vi "Server - Test Inbound Traffic to Server.vi"(8 "error in (no error)":errorcluster, 10 "client address":string="localhost", 11 "ports to check":u16[](array[numeric])=[82, 482, 5672, 6343, 8002, 49580, 22, 44516, 52725, 8080]) -> (0 "error out":errorcluster, 2 "log file path":path, 3 "Results":string[][](array[string]))   [LabVIEW 2019]
doc: "Demonstrates how to open a connection to an TCP server, read the data being sent, and display the data on a chart. This VI is designed to stop if the TCP connection is terminated."
panel:
  out "log file name":string
  out "Current test":cluster{string, "error out":errorcluster}
  in  "Start test":bool
  out "current port":u16
  out "data received":dbl[](graph)
  # "Instructions:\n1. Ensure Client - Test Inbound Traffic to Server is already running.\n2. Run this exe\n3. Click on the button Start Test"
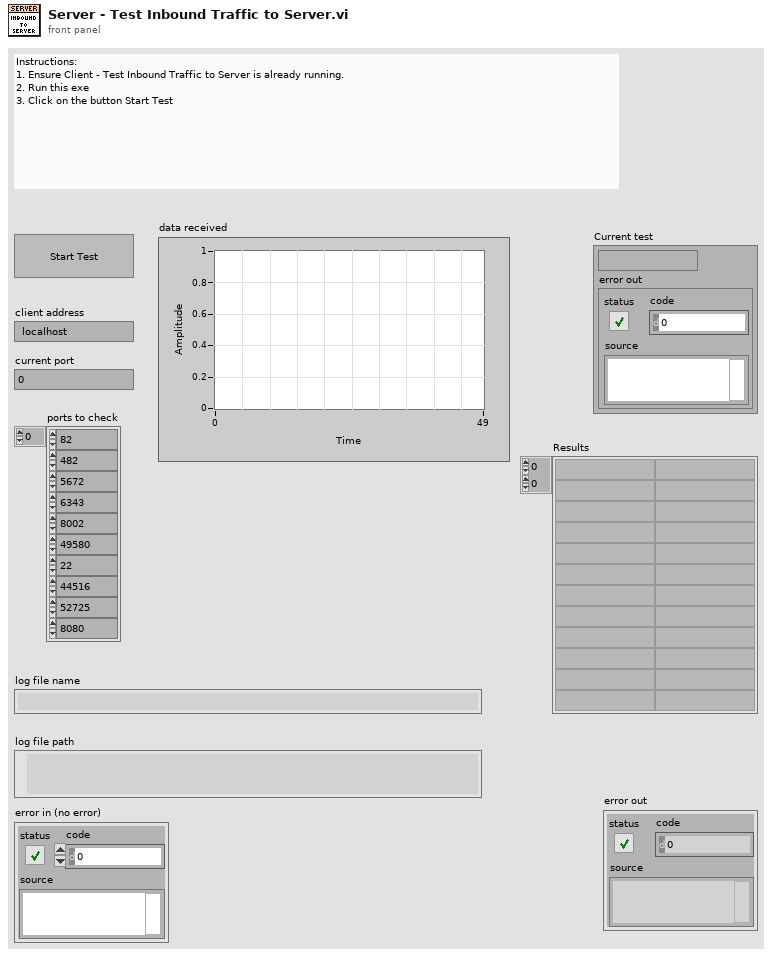
[diagram p1: front panel]
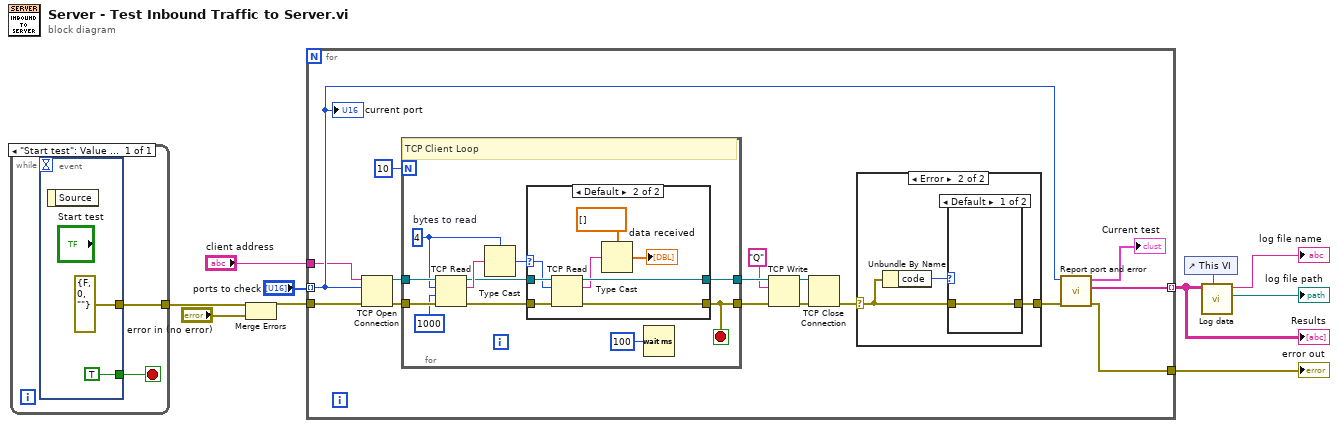
[diagram p0: block diagram]
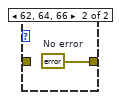
[diagram p4: hidden frame]
diagram:
  n1 = while {
    tunnel: [w12] -> w5
    stop <- w11 stop-if-true
    n2 = event shown="[0] \"Start test\": Value Change" {
      selector: _ -> [_]
      dyn-events: _ -> [_]
      timeout: _ -> [_]
      tunnel: [errorcluster {"status"=FALSE, "code"=0, "source"=""} ("error constant")] -> w12
      tunnel: [TRUE] -> w11
      event "Start test": Value Change {
        n3 = event-data() -> ()  [unwired: 1 in, 1 out]
      }
    }
  }
  n4 = Merge Errors(w5, "error in (no error)") -> (w3:errorcluster)
  n5 = for {
    tunnel: "ports to check" -> [w18] mode=indexing
    tunnel: [w20] -> w10 mode=indexing
    tunnel: w3 -> [w17]
    tunnel: "client address" -> [w16]
    tunnel: [w15] -> w1
    n6 = TCP Open Connection(address=w16, remote port or service name=w18, error in (no error)=w17) -> (connection ID=w30:refnum<k5>, error out=w29:errorcluster)  [unwired: 2 in]
    n7 = for {
      N: 10 -> [_]
      tunnel: w29 -> [w37]
      tunnel: w30 -> [w38]
      tunnel: [w34] -> w27
      tunnel: [w33] -> w25
      stop <- w33 stop-if-true
      w36 = 4  # bytes to read
      # "TCP Client Loop"
      n8 = TCP Read(connection ID=w38, bytes to read=w36, error in (no error)=w37, 9:1000 ("timeout ms (25000)")) -> (connection ID out=w40:refnum<k5>, data out=w41:string, error out=w39:errorcluster)  [unwired: 1 in]
      n9 = Type Cast(type=w36, x=w41) -> (*(type *) &x=w32:i32)
      n10 = case shown="Default" w32 {
        selector: w32 -> [_ w44]
        tunnel: w40 -> [w43 w51]
        tunnel: w39 -> [w42 w50]
        tunnel: [w43 w47] -> w34
        tunnel: [w42 w46] -> w33
        frame ..0 {
          # "The server has not written any data"
        }
        frame Default {
          n11 = TCP Read(connection ID=w51, bytes to read=w44, error in (no error)=w50) -> (connection ID out=w47:refnum<k5>, data out=w45:string, error out=w46:errorcluster)  [unwired: 2 in]
          n12 = Type Cast(type=dbl[] [] ("chart"), x=w45) -> (*(type *) &x=→"data received":dbl[])
        }
      }
      n13 = Wait (ms)(milliseconds to wait=u32 100) -> ()  [unwired: 1 out]
    }
    n14 = TCP Write(connection ID=w27, data in="Q", error in (no error)=w25) -> (connection ID out=w28:refnum<k5>, error out=w26:errorcluster)  [unwired: 2 out]
    n15 = TCP Close Connection(connection ID=w28, error in (no error)=w26) -> (error out=w23:errorcluster)  [unwired: 1 in, 1 out]
    n16 = case shown="Error" w23 {
      selector: w23 -> [w52 w54]
      tunnel: [w52 w53] -> w21
      frame No Error {
      }
      frame Error {
        n17 = Unbundle By Name(w54) -> ("code"=w55:i32)
        n18 = case shown="Default" w55 {
          tunnel: w54 -> [w56 _]
          tunnel: [w56 w57] -> w53
          frame Default {
          }
          frame 62, 64, 66 {
            w57 = errorcluster {"status"=FALSE, "code"=0, "source"=""}  # No error
          }
        }
      }
    }
    n19 = call "Report port and error.vi"("error in (no error)"=w21, "port"=w18) -> ("error out"=w15:errorcluster, "Array"=w20:string[], "output cluster"=→"Current test":cluster{string, "error out":errorcluster})  [unwired: 7 in]
    "current port" <- w18
  }
  "Results" <- w10
  "error out" <- w1
  n20 = control-ref of="This VI"() -> (w7:refnum<vi>)
  n21 = call "Log data.vi"(7:w7, 11:w10) -> ("log file path"=→"log file path":path, "log file name"=→"log file name":string)  [unwired: 7 in, 1 out]
